vi "Autonomous Independent.vi"   [LabVIEW 2013]
doc: "This VI is called when autonomous begins, and will automatically be terminated when autonomous ends. You can carry out timed or sensor driven robot movement independently without needing to return to the caller."
uses:
  <vilib>/Rock Robotics/WPI/Solenoid/WPI_SolenoidValue.ctl
  Robot Global Data.vi
  <vilib>/Rock Robotics/WPI/Solenoid/Deprecated/WPI_SolenoidGetBool.vi
  <vilib>/Rock Robotics/WPI/Solenoid/WPI_SolenoidSetEnum.vi
  <vilib>/Rock Robotics/WPI/RobotDrive/WPI_RobotDriveGetSetRefNum.vi
  <vilib>/Rock Robotics/WPI/RobotDrive/WPI_RobotDriveArcadeDrive_Standard(NoSaturation).vi
  <vilib>/Rock Robotics/WPI/Joystick/WPI_JoystickGetSetRefNum.vi
panel:
  # "Be sure to right-click and choose Data Operations>>Make Current Value default if you want to save the array values with the VI"
types:
  T1 = typedef "WPI_SolenoidDevRef.ctl" = cluster{"DevStatus":errorcluster, "Solenoid Module":T2, "Forward Solenoid Channel":T3, "Reverse Solenoid Channel":T3}
  T2 = typedef "FPGA_TypedefSolenoidModule.ctl" = enum16{"Solenoid Module 1", "Solenoid Module 2"}
  T3 = typedef "WPI_SolenoidChannel.ctl" = enum8{"Solenoid 1", "Solenoid 2", "Solenoid 3", "Solenoid 4", "Solenoid 5", "Solenoid 6", "Solenoid 7", "Solenoid 8", "Invalid"}
  T4 = typedef "WPI_SolenoidValue.ctl" = enum16{"Off", "On", "Forward", "Reverse"}
  T5 = typedef "WPI_RobotDriveDevRef.ctl" = cluster{"DevStatus":errorcluster, "Motors[]":T6[], "Square Inputs":bool, "Max Output":dbl, "Isochronous":bool}
  T6 = typedef "WPI_MotorControlDeviceRef.ctl" = cluster{"DeviceStatus":errorcluster, "Type":enum16{"PWM", "CAN"}, "PWM":cluster{"Digital Module":T7, "PWM Channel":T8, "DeadBand":T9}, "CAN":cluster{"Device Number":u8, "Control Mode":T10, "Semaphore":T11, "Max Vout":dbl}, "Invert":bool, "TransformRef":T12, "InvTransformRef":T12}
  T7 = typedef "FPGA_TypedefDigitalModule.ctl" = enum16{"Digital Module 1", "Digital Module 2"}
  T8 = typedef "FPGA_DIOPWMChannel.ctl" = enum8{"PWM 1", "PWM 2", "PWM 3", "PWM 4", "PWM 5", "PWM 6", "PWM 7", "PWM 8", "PWM 9", "PWM 10", "Invalid"}
  T9 = typedef "WPI_PWMDeadband.ctl" = cluster{"Name":string, "maxPositivePwm":i32, "minPositivePwm":i32, "centerPwm":i32, "maxNegativePwm":i32, "minNegativePwm":i32, "angularRange":u16}
  T10 = typedef "WPI_CANJaguar_ControlMode.ctl" = enum8{"Percent VBus", "Current", "Speed", "Position", "Voltage"}
  T11 = typedef "Semaphore RefNum" = refnum<k1>
  T12 = typedef "WPI_PWMTransform_ConPane.ctl" = refnum<vi>
  T13 = typedef "WPI_JoystickDevRef.ctl" = cluster{"Device":T14}
  T14 = typedef "WPI_JoystickDeviceEnum.ctl" = enum16{"USB 1", "USB 2", "USB 3", "USB 4", "Kinect 1", "Kinect 2"}
  T15 = cluster{"axis 1 (x)":dbl, "axis 2 (y)":dbl, "axis 3 (throttle)":dbl, "axis 4":dbl, "axis 5":dbl, "axis 6":dbl}
  T16 = typedef "WPI_DigitalInputDevRef.ctl" = cluster{"DevStatus":errorcluster, "DIO Channel":T17, "Digital Module":T7}
  T17 = typedef "FPGA_DIOChannel.ctl" = enum8{"DIO 1", "DIO 2", "DIO 3", "DIO 4", "DIO 5", "DIO 6", "DIO 7", "DIO 8", "DIO 9", "DIO 10", "DIO 11", "DIO 12", "DIO 13", "DIO 14", "Invalid"}
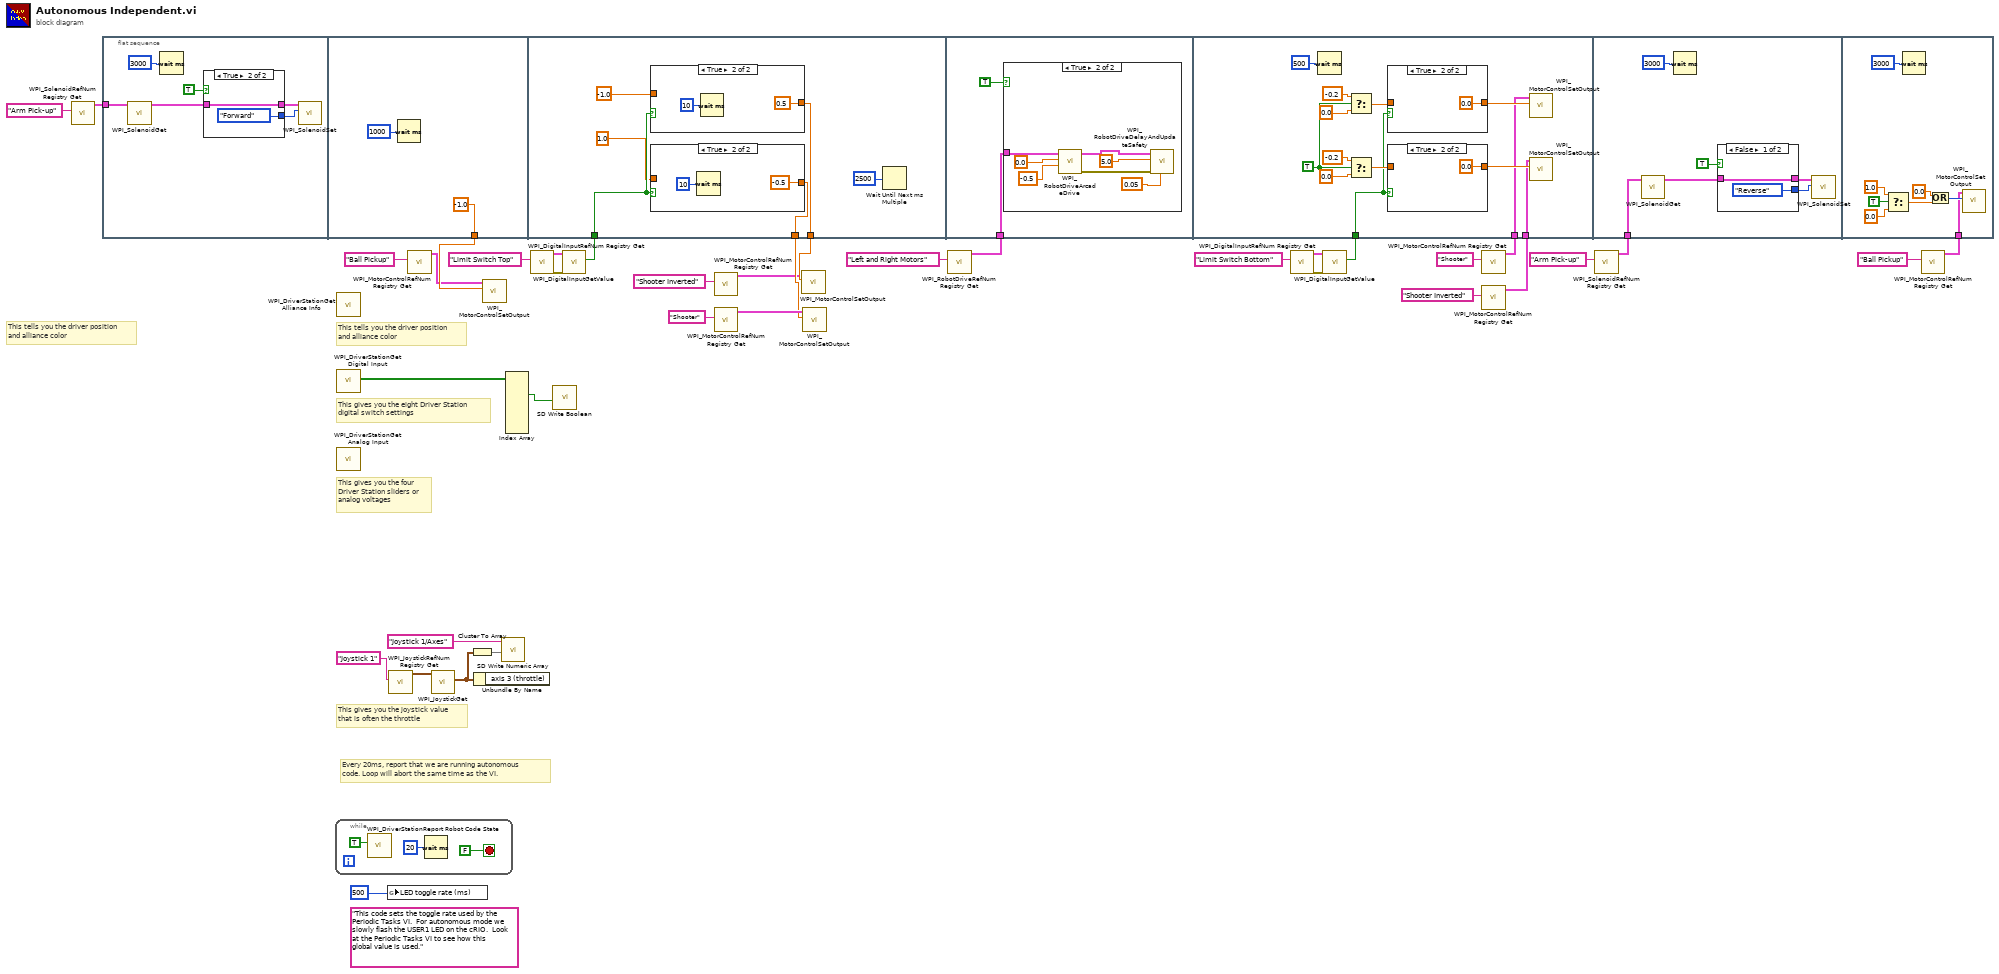
[diagram p0: block diagram]
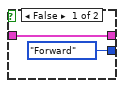
[diagram p2: hidden frame]
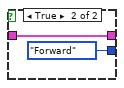
[diagram p8: hidden frame]
diagram:
  (unwired) "This code sets the toggle rate used by the Periodic Tasks VI.  For autonomous mode we slowly flash the USER1 LED on the cRIO.  Look at the Periodic Tasks VI to see how this global value is used."
  # "This tells you the driver position\nand alliance color"
  # "Every 20ms, report that we are running autonomous\ncode. Loop will abort the same time as the VI."
  # "This gives you the joystick value\nthat is often the throttle"
  # "This tells you the driver position\nand alliance color"
  # "This gives you the eight Driver Station\ndigital switch settings"
  # "This gives you the four\nDriver Station sliders or\nanalog voltages"
  n1 = call <vilib>:"WPI_SolenoidRefNum Registry Get.vi"("refnum name"="Arm Pick-up") -> ("SolenoidDevRef"=w15:T1)  [unwired: 9 in, 1 out]
  n2 = flat-sequence {
    tunnel: w15 -> [w38]
    tunnel: [-1.0 ("Output")] -> w6
    tunnel: w21 -> [w55]
    tunnel: [w52] -> w4
    tunnel: [w51] -> w2
    tunnel: w20 -> [w62]
    tunnel: w25 -> [w73]
    tunnel: w13 -> [w72]
    tunnel: w11 -> [w71]
    tunnel: w9 -> [w88]
    tunnel: w7 -> [w98]
    frame #0 {
      n3 = call-poly <vilib>:"WPI_SolenoidGet.vi"("SolenoidDevRef"=w38) -> ("SolenoidDevRef"=w43:T1)  [unwired: 8 in, 2 out]
      n4 = Wait (ms)(milliseconds to wait=u32 3000) -> ()  [unwired: 1 out]
      n5 = case shown="True" TRUE {
        tunnel: w43 -> [w44 w47]
        tunnel: [w44 w47] -> w42
        tunnel: [WPI_SolenoidValue."Forward" ("Value") WPI_SolenoidValue."Forward" ("Value")] -> w41
        frame False {
        }
        frame True {
        }
      }
      n6 = call-poly <vilib>:"WPI_SolenoidSet.vi"("Value"=w41, "SolenoidDevRef"=w42) -> ()  [unwired: 8 in, 2 out]
    }
    frame #1 {
      n7 = Wait (ms)(milliseconds to wait=u32 1000) -> ()  [unwired: 1 out]
    }
    frame #2 {
      n8 = case shown="True" w55 {
        tunnel: [w56 0.5 ("f")] -> w52
        tunnel: -1.0 ("t") -> [w56 _]
        frame False {
        }
        frame True {
          n9 = Wait (ms)(milliseconds to wait=u32 10) -> ()  [unwired: 1 out]
        }
      }
      n10 = case shown="True" w55 {
        tunnel: [w59 -0.5 ("f")] -> w51
        tunnel: 1.0 ("t") -> [w59 _]
        frame False {
        }
        frame True {
          n11 = Wait (ms)(milliseconds to wait=u32 10) -> ()  [unwired: 1 out]
        }
      }
      n12 = Wait Until Next ms Multiple(millisecond multiple=u32 2500) -> ()  [unwired: 1 out]
    }
    frame #3 {
      n13 = case shown="True" TRUE {
        tunnel: w62 -> [_ w70]
        frame False {
        }
        frame True {
          n14 = call-poly <vilib>:"WPI_RobotDriveArcadeDrive.vi"("Y axis value"=-0.5, "X axis value"=0.0, "RobotDriveDevRef"=w70) -> ("error out"=w67:errorcluster, "RobotDriveDevRef"=w66:T5)  [unwired: 6 in, 1 out]
          n15 = call <vilib>:"WPI_RobotDriveDelayAndUpdateSafety.vi"("Feed time (s)"=0.05, "error in (no error)"=w67, "Delay (s)"=5.0, "RobotDriveDevRef"=w66) -> ()  [unwired: 6 in, 2 out]
        }
      }
    }
    frame #4 {
      w74 = TRUE
      n16 = Wait (ms)(milliseconds to wait=u32 500) -> ()  [unwired: 1 out]
      n17 = Select(t=-0.2, s=w74, f=0.0) -> (s? t:f=w76:dbl)
      n18 = Select(t=-0.2, s=w74, f=0.0) -> (s? t:f=w75:dbl)
      n19 = case shown="True" w73 {
        tunnel: [w86 0.0 ("f")] -> w81
        tunnel: w76 -> [w86 _]
        frame False {
        }
        frame True {
        }
      }
      n20 = case shown="True" w73 {
        tunnel: [w84 0.0 ("f")] -> w78
        tunnel: w75 -> [w84 _]
        frame False {
        }
        frame True {
        }
      }
      n21 = call <vilib>:"WPI_MotorControlSetOutput.vi"("Output"=w81, "MotorControlDevRef"=w71) -> ()  [unwired: 7 in, 3 out]
      n22 = call <vilib>:"WPI_MotorControlSetOutput.vi"("Output"=w78, "MotorControlDevRef"=w72) -> ()  [unwired: 7 in, 3 out]
    }
    frame #5 {
      n23 = call-poly <vilib>:"WPI_SolenoidGet.vi"("SolenoidDevRef"=w88) -> ("SolenoidDevRef"=w93:T1)  [unwired: 8 in, 2 out]
      n24 = Wait (ms)(milliseconds to wait=u32 3000) -> ()  [unwired: 1 out]
      n25 = case shown="False" TRUE {
        tunnel: w93 -> [w94 w97]
        tunnel: [w94 w97] -> w92
        tunnel: [WPI_SolenoidValue."Reverse" ("Value") WPI_SolenoidValue."Forward" ("Value")] -> w91
        frame False {
        }
        frame True {
        }
      }
      n26 = call-poly <vilib>:"WPI_SolenoidSet.vi"("Value"=w91, "SolenoidDevRef"=w92) -> ()  [unwired: 8 in, 2 out]
    }
    frame #6 {
      n27 = Select(t=1.0, s=TRUE, f=0.0) -> (s? t:f=w102:dbl)
      n28 = Wait (ms)(milliseconds to wait=u32 3000) -> ()  [unwired: 1 out]
      n29 = Or(x=0.0, y=w102) -> (x .or. y?=w101:i32)
      n30 = call <vilib>:"WPI_MotorControlSetOutput.vi"("Output"=w101, "MotorControlDevRef"=w98) -> ()  [unwired: 7 in, 3 out]
    }
  }
  n31 = while {
    stop <- FALSE stop-if-true
    n32 = call <vilib>:"WPI_DriverStationReport Robot Code State.vi"("Autonomous"=TRUE) -> ()  [unwired: 10 in, 1 out]
    n33 = Wait (ms)(milliseconds to wait=u32 20) -> ()  [unwired: 1 out]
  }
  n34 = call <vilib>:"WPI_DriverStationGet Alliance Info.vi"() -> ()  [unwired: 12 out]
  n35 = call <vilib>:"WPI_DriverStationGet Digital Input.vi"() -> ("Driver Station Digital Input (1-8)"=w37:bool[])  [unwired: 11 out]
  n36 = call <vilib>:"WPI_DriverStationGet Analog Input.vi"() -> ()  [unwired: 12 out]
  n37 = global write "Robot Global Data.vi" "LED toggle rate (ms)"(u32 500 ("LED ms toggle rate")) -> ()
  n38 = call <vilib>:"WPI_JoystickRefNum Registry Get.vi"("refnum name"="Joystick 1") -> ("JoystickDevRef"=w35:T13)  [unwired: 1 in, 9 out]
  n39 = call <vilib>:"WPI_MotorControlRefNum Registry Get.vi"("refnum name"="Ball Pickup") -> ("MotorControlDevRef"=w5:T6)  [unwired: 9 in, 1 out]
  n40 = call <vilib>:"WPI_JoystickGet.vi"("JoystickDevRef"=w35) -> ("Axes"=w32:T15)  [unwired: 1 in, 5 out]
  n41 = Cluster To Array(cluster=w32) -> (array=w33:dbl[])
  n42 = Unbundle By Name(w32) -> ()  [unwired: 1 out]
  n43 = call <vilib>:"WPI_MotorControlSetOutput.vi"("Output"=w6, "MotorControlDevRef"=w5) -> ()  [unwired: 7 in, 3 out]
  n44 = call <vilib>:"SD Write Numeric Array.vi"("Numeric Array"=w33, "Name"="Joystick 1/Axes") -> ()  [unwired: 8 in, 2 out]
  n45 = Index Array(array=w37) -> (element #2=w30:bool)  [unwired: 8 in, 7 out]
  n46 = call <vilib>:"WPI_DigitalInputRefNum Registry Get.vi"("refnum name"="Limit Switch Top") -> ("error out"=w23:errorcluster, "DigitalInputDevRef"=w24:T16)  [unwired: 9 in]
  n47 = call <vilib>:"SD Write Boolean.vi"("Boolean"=w30) -> ()  [unwired: 9 in, 2 out]
  n48 = call <vilib>:"WPI_DigitalInputGetValue.vi"("error in (no error)"=w23, "DigitalInputDevRef"=w24) -> ("Value"=w21:bool)  [unwired: 7 in, 2 out]
  n49 = call <vilib>:"WPI_MotorControlRefNum Registry Get.vi"("refnum name"="Shooter Inverted") -> ("MotorControlDevRef"=w1:T6)  [unwired: 9 in, 1 out]
  n50 = call <vilib>:"WPI_MotorControlRefNum Registry Get.vi"("refnum name"="Shooter") -> ("MotorControlDevRef"=w3:T6)  [unwired: 9 in, 1 out]
  n51 = call <vilib>:"WPI_MotorControlSetOutput.vi"("Output"=w4, "MotorControlDevRef"=w1) -> ()  [unwired: 7 in, 3 out]
  n52 = call <vilib>:"WPI_MotorControlSetOutput.vi"("Output"=w2, "MotorControlDevRef"=w3) -> ()  [unwired: 7 in, 3 out]
  n53 = call <vilib>:"WPI_RobotDriveRefNum Registry Get.vi"("refnum name"="Left and Right Motors") -> ("RobotDriveDevRef"=w20:T5)  [unwired: 9 in, 1 out]
  n54 = call <vilib>:"WPI_DigitalInputRefNum Registry Get.vi"("refnum name"="Limit Switch Bottom") -> ("error out"=w27:errorcluster, "DigitalInputDevRef"=w28:T16)  [unwired: 9 in]
  n55 = call <vilib>:"WPI_DigitalInputGetValue.vi"("error in (no error)"=w27, "DigitalInputDevRef"=w28) -> ("Value"=w25:bool)  [unwired: 7 in, 2 out]
  n56 = call <vilib>:"WPI_MotorControlRefNum Registry Get.vi"("refnum name"="Shooter") -> ("MotorControlDevRef"=w11:T6)  [unwired: 9 in, 1 out]
  n57 = call <vilib>:"WPI_MotorControlRefNum Registry Get.vi"("refnum name"="Shooter Inverted") -> ("MotorControlDevRef"=w13:T6)  [unwired: 9 in, 1 out]
  n58 = call <vilib>:"WPI_SolenoidRefNum Registry Get.vi"("refnum name"="Arm Pick-up") -> ("SolenoidDevRef"=w9:T1)  [unwired: 9 in, 1 out]
  n59 = call <vilib>:"WPI_MotorControlRefNum Registry Get.vi"("refnum name"="Ball Pickup") -> ("MotorControlDevRef"=w7:T6)  [unwired: 9 in, 1 out]
